vi "dB To Amplitude.vi"(11 "dB":dbl) -> (3 "Amplitude":dbl)   [LabVIEW 2019, in "Audio Processing.lvlib"]
doc: "Convert the decibel value into amplitude."
uses:
  Audio Processing.lvlib
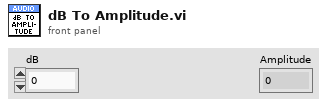
[diagram p1: front panel]
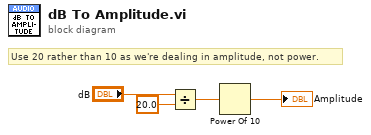
[diagram p0: block diagram]
diagram:
  # "Use 20 rather than 10 as we're dealing in amplitude, not power."
  n1 = Divide(x="dB", y=20.0) -> (x/y=w2:dbl)
  n2 = Power Of 10(x=w2) -> (10^x=→"Amplitude":dbl)
